vi "2,4,6,8 ON.vi"() -> ()   [LabVIEW 2017]
panel:
  out "x=8":bool
  out "x = 6":bool
  out "x =4":bool
  out "x = 2":bool
  out "x":i32
  out "interaction":i32
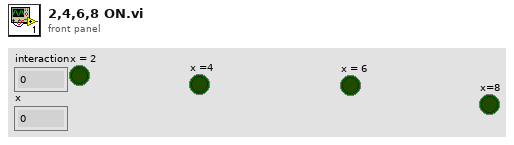
[diagram p1: front panel]
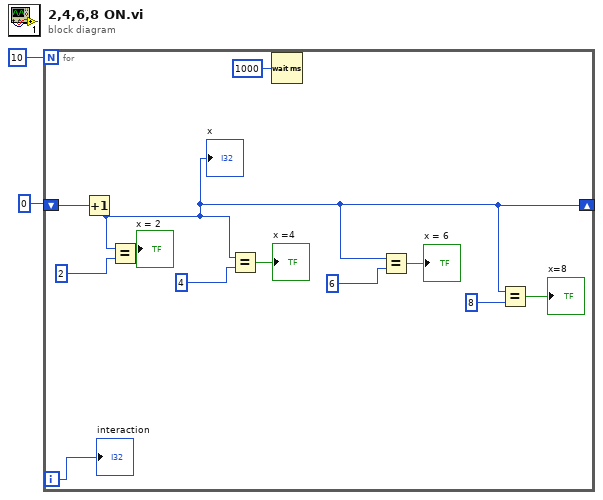
[diagram p0: block diagram]
diagram:
  n1 = for {
    N: 10 -> [_]
    shift-right: [w4] -> _
    shift-left: 0 -> [w13]
    i -> [w14]
    n2 = Increment(x=w13) -> (x+1=w4:i32)
    "x" <- w4
    n3 = Equal?(x=w4, y=2) -> (x = y?=→"x = 2":bool)
    n4 = Equal?(x=w4, y=4) -> (x = y?=→"x =4":bool)
    n5 = Wait (ms)(milliseconds to wait=u32 1000) -> ()  [unwired: 1 out]
    n6 = Equal?(x=w4, y=6) -> (x = y?=→"x = 6":bool)
    n7 = Equal?(x=w4, y=8) -> (x = y?=→"x=8":bool)
    "interaction" <- w14
  }
